vi "被反馈处理-修改内容.vi"(1 "反馈无CRCU8数组":u8[](array[numeric])) -> (15 "反馈":string)   [LabVIEW 2019]
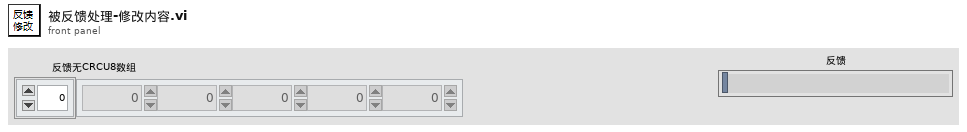
[diagram p1: front panel]
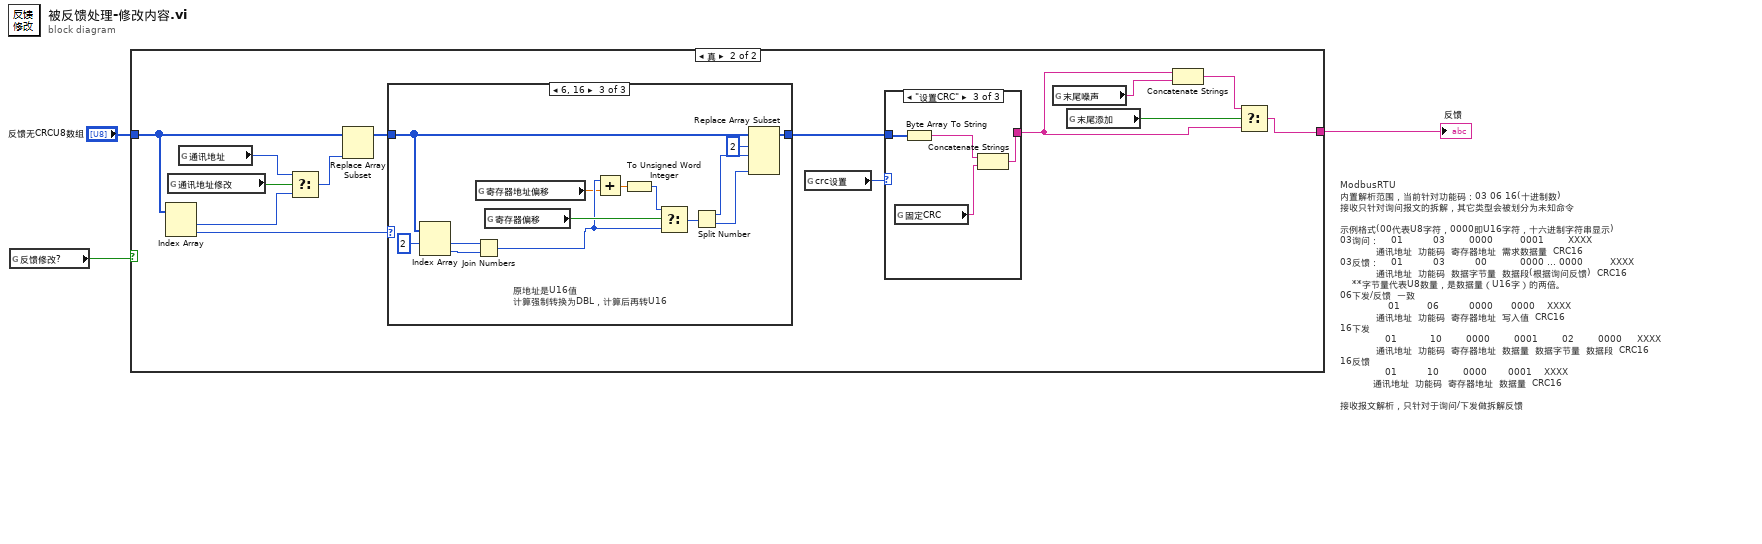
[diagram p0: block diagram]
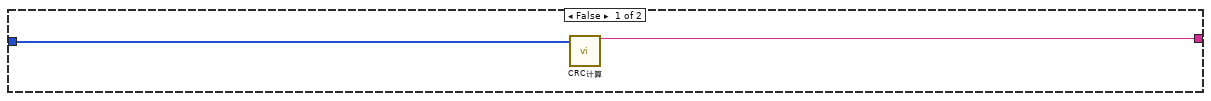
[diagram p2: hidden frame]
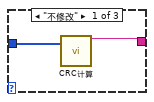
[diagram p3: hidden frame]
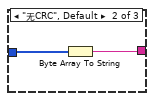
[diagram p4: hidden frame]
diagram:
  # "ModbusRTU\n内置解析范围，当前针对功能码：03 06 16(十进制数)\n接收只针对询问报文的拆解，其它类型会被划分为未知命令\n\n示例格式(00代表U8字符，0000即U16字符，十六进制字符串显示)\n03询问：    01          03        0000         0001        XXXX \n            通讯地址  功能码  寄存器地址  需求数据量  CRC16\n03反馈：    01          03          00           0000 ... 0000         XXXX \n            通讯地址  功能码  数据字节量  数据段(根据询问反馈)  CRC16\n    **字节量代表U8数量，是数据量（U16字）的两倍。\n06下发/反馈  一致\n                01         06          0000      0000    XXXX\n            通讯地址  功能码  寄存器地址  写入值  CRC16\n16下发\n               01           10        0000        0001        02        0000     XXXX\n            通讯地址  功能码  寄存器地址  数据量  数据字节量  数据段  CRC16 \n16反馈\n               01          10        0000       0001    XXXX\n           通讯地址  功能码  寄存器地址  数据量  CRC16\n\n接收报文解析，只针对于询问/下发做拆解反馈"
  n1 = global read "全局-被反馈配置.vi" "反馈修改?"() -> (w1:bool)
  n2 = case shown="真" w1 {
    tunnel: "反馈无CRCU8数组" -> [w5 w18]
    tunnel: [w4 w6] -> w2
    frame False {
      n3 = call "CRC计算.vi"("无校验U8数组"=w5) -> ("计算后字符串"=w4:string)  [unwired: 17 in, 1 out]
    }
    frame True {
      n4 = Index Array(array=w18) -> (element #1=w15:u8, element #2=w19:u8)  [unwired: 2 in]
      n5 = global read "全局-被反馈配置.vi" "通讯地址修改"() -> (w16:bool)
      n6 = global read "全局-被反馈配置.vi" "通讯地址"() -> (w14:u8)
      n7 = Select(t=w14, s=w16, f=w15) -> (s? t:f=w13:u8)
      n8 = Replace Array Subset(array=w18, new element=w13) -> (w17:u8[])  [unwired: 1 in]
      n9 = case shown="6, 16" w19 {
        tunnel: w17 -> [w28 w29 w33]
        tunnel: [w28 w29 w30] -> w12
        frame Default {
        }
        frame 3 {
        }
        frame 6, 16 {
          # "原地址是U16值\n计算强制转换为DBL，计算后再转U16"
          n10 = Index Array(array=w33, index #1=2 ("索引")) -> (element #1=w42:u8, element #2=w41:u8)  [unwired: 1 in]
          n11 = Join Numbers(hi=w42, lo=w41) -> ((hi.lo)=w39:u16)
          n12 = global read "全局-被反馈配置.vi" "寄存器地址偏移"() -> (w38:dbl)
          n13 = global read "全局-被反馈配置.vi" "寄存器偏移"() -> (w40:bool)
          n14 = Add(x=w39, y=w38) -> (x+y=w37:dbl)
          n15 = To Unsigned Word Integer(number=w37) -> (unsigned 16bit integer=w36:u16)
          n16 = Select(t=w36, s=w40, f=w39) -> (s? t:f=w35:u16)
          n17 = Split Number(x=w35) -> (hi(x)=w32:u8, lo(x)=w31:u8)
          n18 = Replace Array Subset(array=w33, new element #1=w32, index #1=2 ("索引"), new element #2=w31) -> (w30:u8[])  [unwired: 1 in]
        }
      }
      n19 = global read "全局-被反馈配置.vi" "crc设置"() -> (w11:enum32{"不修改", "无CRC", "设置CRC"})
      n20 = case shown="\"设置CRC\"" w11 {
        tunnel: w12 -> [w21 w23 w27]
        tunnel: [w20 w22 w24] -> w9
        frame "不修改" {
          n21 = call "CRC计算.vi"("无校验U8数组"=w21) -> ("计算后字符串"=w20:string)  [unwired: 17 in, 1 out]
        }
        frame "无CRC", Default {
          n22 = Byte Array To String(unsigned byte array=w23) -> (string=w22:string)
        }
        frame "设置CRC" {
          n23 = global read "全局-被反馈配置.vi" "固定CRC"() -> (w25:string)
          n24 = Byte Array To String(unsigned byte array=w27) -> (string=w26:string)
          n25 = Concatenate Strings(w26, w25) -> (w24:string)
        }
      }
      n26 = global read "全局-被反馈配置.vi" "末尾噪声"() -> (w8:string)
      n27 = global read "全局-被反馈配置.vi" "末尾添加"() -> (w10:bool)
      n28 = Concatenate Strings(w9, w8) -> (w7:string)
      n29 = Select(t=w7, s=w10, f=w9) -> (s? t:f=w6:string)
    }
  }
  "反馈" <- w2
